vi "Add Protection.vi"(8 "error in (no error)":errorcluster, 9 "Pad":bool, 10 "String in":string, 11 "Checksum U32 in":refnum<class "Checksum U32.lvclass">) -> (0 "error out":errorcluster, 2 "String out":string, 3 "Checksum U32 out":refnum<class "Checksum U32.lvclass">)   [LabVIEW 2019, in "Protections.lvlib" / "Checksum U32.lvclass"]
uses:
  Checksum U32.lvclass
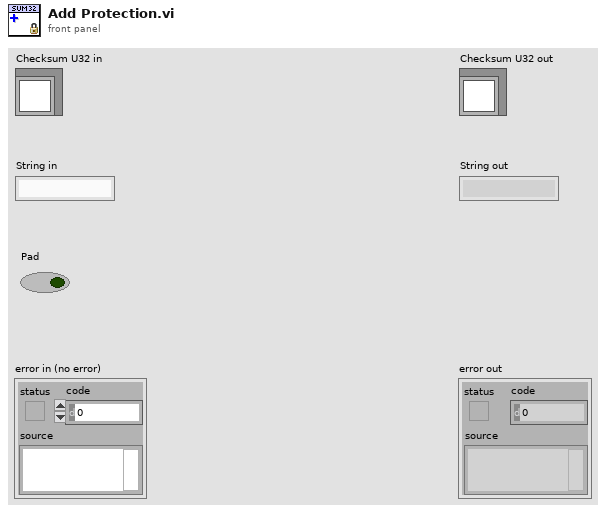
[diagram p1: front panel]
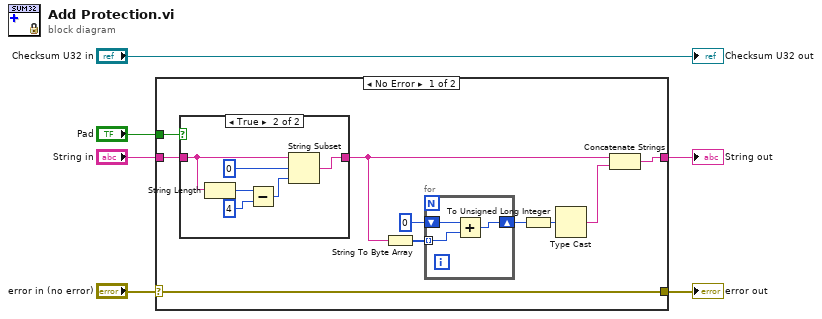
[diagram p0: block diagram]
diagram:
  n1 = case shown="No Error" "error in (no error)" {
    selector: "error in (no error)" -> [w10 w28]
    tunnel: "Pad" -> [w7 _]
    tunnel: "String in" -> [w9 w27]
    tunnel: [w11 w27] -> w1
    tunnel: [w10 w28] -> w6
    frame No Error {
      n2 = case shown="True" w7 {
        tunnel: w9 -> [w17 w23]
        tunnel: [w17 w18] -> w8
        frame False {
        }
        frame True {
          n3 = String Length(string=w23) -> (length=w21:i32)
          n4 = Subtract(x=w21, y=4) -> (x-y=w19:i32)
          n5 = String Subset(string=w23, offset (0)=0, length (rest)=w19) -> (substring=w18:string)
        }
      }
      n6 = String To Byte Array(string=w8) -> (unsigned byte array=w16:u8[])
      n7 = for {
        tunnel: w16 -> [w26] mode=indexing
        shift-right: [w24] -> w14
        shift-left: u64 0 -> [w25]
        n8 = Add(x=w25, y=w26) -> (x+y=w24:u64)
      }
      n9 = To Unsigned Long Integer(number=w14) -> (unsigned 32bit integer=w12:u32)
      n10 = Type Cast(x=w12) -> (*(type *) &x=w13:string)  [unwired: 1 in]
      n11 = Concatenate Strings(w8, w13) -> (w11:string)
    }
    frame Error {
    }
  }
  "error out" <- w6
  "String out" <- w1
  "Checksum U32 out" <- "Checksum U32 in"
